vi "160-Inner Test.vi"(8 "error in (no error)":errorcluster, 11 "Label (VI Title)":string="Inner Test") -> (0 "error out":errorcluster)   [LabVIEW 2013]
uses:
  classes/Assert/Assert True.vi
  classes/Test/Test.lvclass
  classes/Assert/Assert.lvclass
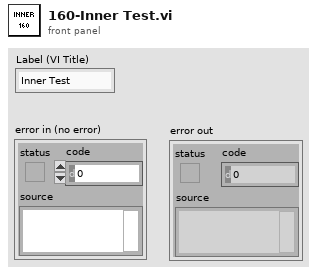
[diagram p1: front panel]
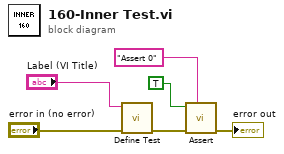
[diagram p0: block diagram]
diagram:
  n1 = call "Define Test.vi"("error in (no error)"="error in (no error)", "Label (VI Title)"="Label (VI Title)") -> ("error out"=w5:errorcluster)  [unwired: 8 in, 1 out]
  n2 = call-poly "Assert.vi"("Label"="Assert 0", "error in (no error)"=w5, "True?"=TRUE) -> ("error out"=→"error out":errorcluster)  [unwired: 7 in, 1 out]
